vi "lookup_node_by_id_array.vi"(10 "node_ids":refnum<class "ID.lvclass">[](array[class]), 11 "graph":refnum<class "Graph.lvclass">) -> (1 "nodes":refnum<class "Node.lvclass">[](array[class]), 2 "any nodes not found?":bool)   [LabVIEW 2020, in "graph.lvlib" / "Graph.lvclass"]
uses:
  Graph.lvclass
  ID/ID.lvclass
  Node/Node.lvclass
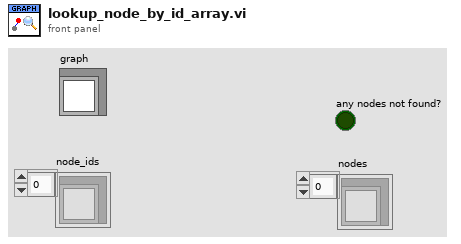
[diagram p1: front panel]
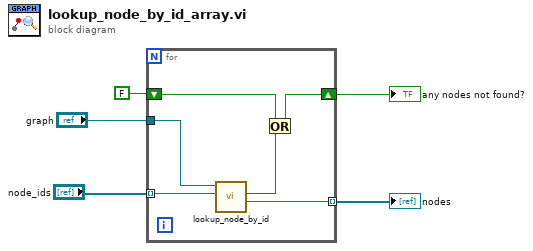
[diagram p0: block diagram]
diagram:
  n1 = for {
    tunnel: "node_ids" -> [w10] mode=indexing
    tunnel: [w9] -> w1 mode=indexing
    tunnel: "graph" -> [w11]
    shift-right: [w6] -> w2
    shift-left: FALSE -> [w7]
    n2 = call "lookup_node_by_id.vi"("node_id"=w10, "graph"=w11) -> ("node"=w9:refnum<class "Node.lvclass">, "node not found?"=w8:bool)  [unwired: 8 in]
    n3 = Or(x=w7, y=w8) -> (x .or. y?=w6:bool)
  }
  "nodes" <- w1
  "any nodes not found?" <- w2
